vi "Sub Initialize.vi"(8 "error in (no error)":errorcluster, 11 "Instrument Recorder in":refnum<class "Instrument Actor.lvclass">) -> (0 "error out":errorcluster, 2 "Initialize Result":refnum<class "Acquired Result.lvclass">, 3 "Instrument Recorder out":refnum<class "Instrument Actor.lvclass">)   [LabVIEW 2016, in "Instrument Actor.lvclass"]
uses:
  Instrument Actor.lvclass
  C:/github/LabActor/Template Module/Template Module.lvclass
  C:/github/LabActor/Worker/Worker.lvclass
  Results/Acquired Result/Acquired Result.lvclass
  Instrument Actor.lvclass/Instrument Actor.ctl
  Template Module/Template Module.lvclass/Template Module.ctl
  Worker/Worker.lvclass/Worker.ctl
  NHMFL_Core/Libraries/Instruments/Instrument Driver/Instrument Driver.lvclass/Instrument Driver.ctl
  Read Instrument driver.vi
  Template Module/Read Configuration.vi
  Template Module/Read Name.vi
  Worker/Read Cycle period.vi
  NHMFL_Core/Libraries/Instruments/Instrument Driver/Write Recorder name.vi
  NHMFL_Core/Libraries/Instruments/Instrument Driver/Write Cycle period.vi
  Write Instrument driver.vi
  NHMFL_Core/Libraries/Instruments/Instrument Driver/Write User configuration.vi
  NHMFL_Core/Libraries/Instruments/Instrument Driver/Instrument Driver.lvclass
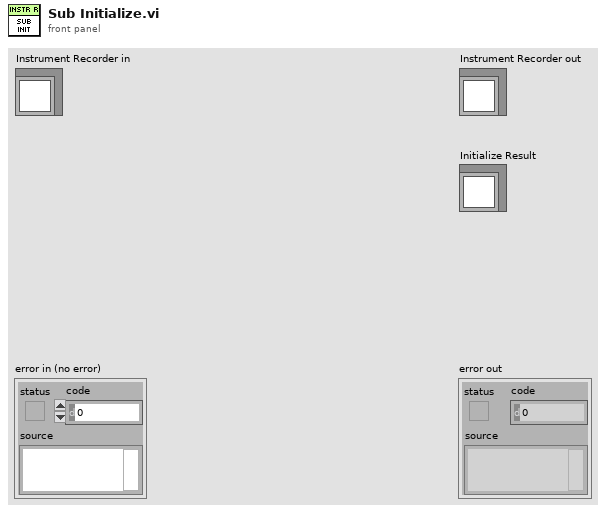
[diagram p1: front panel]
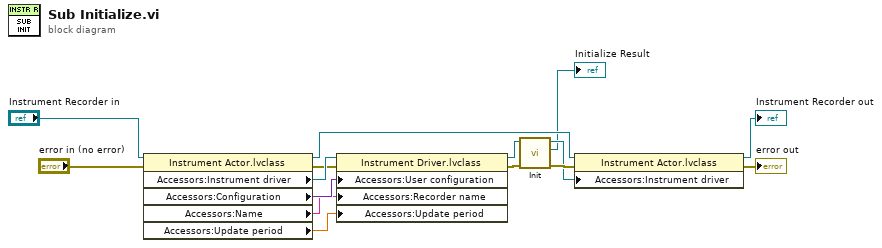
[diagram p0: block diagram]
diagram:
  n1 = property class="Instrument Actor.lvclass"(reference="Instrument Recorder in", error in="error in (no error)") -> (reference out=w14:refnum<class "Instrument Actor.lvclass">, error out=w4:errorcluster, "Accessors:Instrument driver"=w7:refnum<class "Instrument Driver.lvclass">, "Accessors:Configuration"=w5:variant, "Accessors:Name"=w2:string, "Accessors:Update period"=w1:dbl)
  n2 = property class="Instrument Driver.lvclass"(reference=w7, error in=w4, "Accessors:User configuration"=w5, "Accessors:Recorder name"=w2, "Accessors:Update period"=w1) -> (reference out=w6:refnum<class "Instrument Driver.lvclass">, error out=w3:errorcluster)
  n3 = call-dynamic "Init.vi"("error in (no error)"=w3, "Instrument Driver in"=w6) -> ("error out"=w12:errorcluster, "Init Result"=→"Initialize Result":refnum<class "Acquired Result.lvclass">, "Instrument Driver out"=w11:refnum<class "Instrument Driver.lvclass">)  [unwired: 7 in]
  n4 = property class="Instrument Actor.lvclass"(reference=w14, error in=w12, "Accessors:Instrument driver"=w11) -> (reference out=→"Instrument Recorder out":refnum<class "Instrument Actor.lvclass">, error out=→"error out":errorcluster)
